vi "Cancel State Machine - Polymorphic.vi"   [LabVIEW 2013]
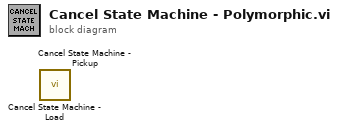
[diagram p0: block diagram]
diagram:
  n1 = call "Cancel State Machine - Load.vi"() -> ()  [unwired: 1 in]
  n2 = call "Cancel State Machine - Pickup.vi"() -> ()  [unwired: 1 in]
